vi "Get Record Length.vi"(7 "instance":i32, 8 "error in":errorcluster, 11 "lia host in":refnum<class "LIA Host Interface FPGA.lvclass">) -> (0 "error out":errorcluster, 2 "record length":u32, 3 "lia host out":refnum<class "LIA Host Interface FPGA.lvclass">)   [LabVIEW 2017, in "LIA Host Interface FPGA.lvclass"]
uses:
  LIA Host Interface FPGA.lvclass
  LIA Host Interface FPGA.lvclass/LIA Host Interface FPGA.ctl
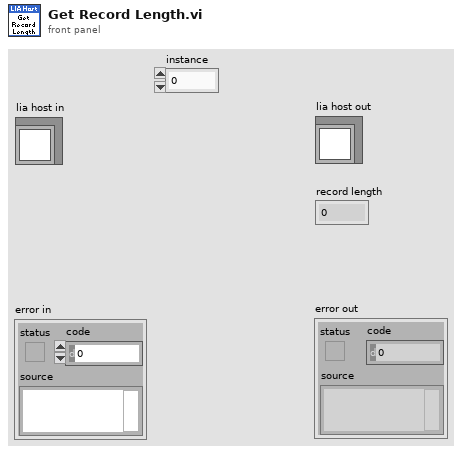
[diagram p1: front panel]
types:
  T1 = typedef "LIA Host Interface Desktop.lvclass/session data.ctl" = cluster{"fpga session":refnum<k20>, "record length":u32[]}
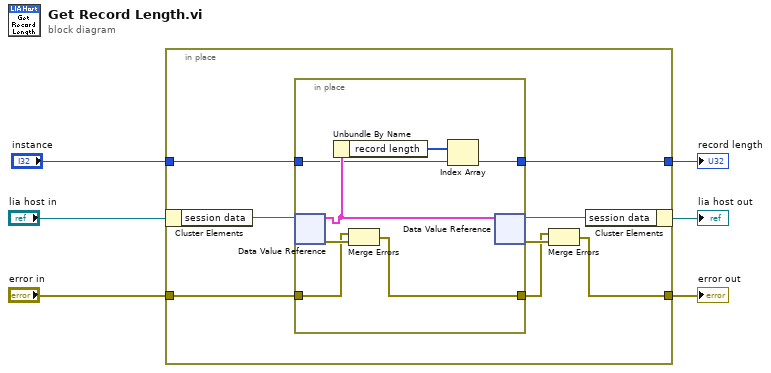
[diagram p0: block diagram]
diagram:
  n1 = in-place {
    in-place-border: "error in" -> [w12]
    in-place-border: [w9] -> w3
    in-place-border: "instance" -> [w8]
    in-place-border: [w7] -> w1
    n2 = in-place-cluster #1("lia host in") -> ("session data"=w14:refnum<data-value>)
    n3 = in-place {
      in-place-border: w12 -> [w20]
      in-place-border: [w19] -> w10
      in-place-border: w8 -> [w16]
      in-place-border: [w15] -> w7
      n4 = in-place-dvr #2(w14) -> (w18:T1, w21:errorcluster)
      n5 = Unbundle By Name(w18) -> ("record length"=w17:u32[])
      n6 = Merge Errors(w20, w21) -> (w19:errorcluster)
      n7 = Index Array(array=w17, index=w16) -> (element=w15:u32)
      n8 = in-place-dvr #2(w18) -> (w13:refnum<data-value>, w11:errorcluster)
    }
    n9 = Merge Errors(w10, w11) -> (w9:errorcluster)
    n10 = in-place-cluster #1("session data"=w13) -> (→"lia host out":refnum<class "LIA Host Interface FPGA.lvclass">)
  }
  "error out" <- w3
  "record length" <- w1
